vi "Dictionary.Compare.vi"(8 "error in (no error)":errorcluster, 10 "Original Data (Dictionary)":T1[](array[typedef]), 11 "Converted Data (Dictionary)":T1[](array[typedef])) -> (0 "error out":errorcluster, 3 "Not Equal?":bool)   [LabVIEW 2019, in "Conversion.lvclass"]
uses:
  Conversion.lvclass
  _OpenG.lib/numeric/numeric.llb/Random Number Within Range - I32__ogtk.vi
  Data/Typedefs/Dictionary--cluster.ctl
  Data/Data.lvclass
panel:
  out "element":string
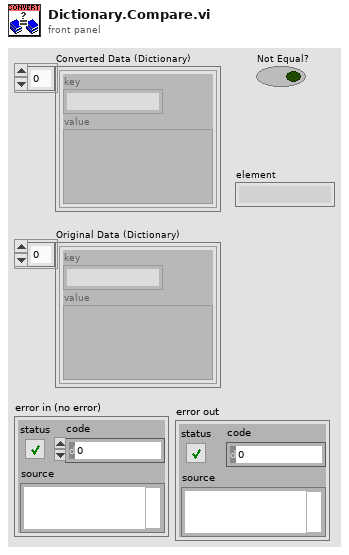
[diagram p1: front panel]
types:
  T1 = typedef "Data.lvclass/Dictionary--cluster.ctl" = cluster{"key":string, "value":variant}
  T2 = typedef "Dictionary Object RefNum__ogtk.ctl" = refnum<k1>
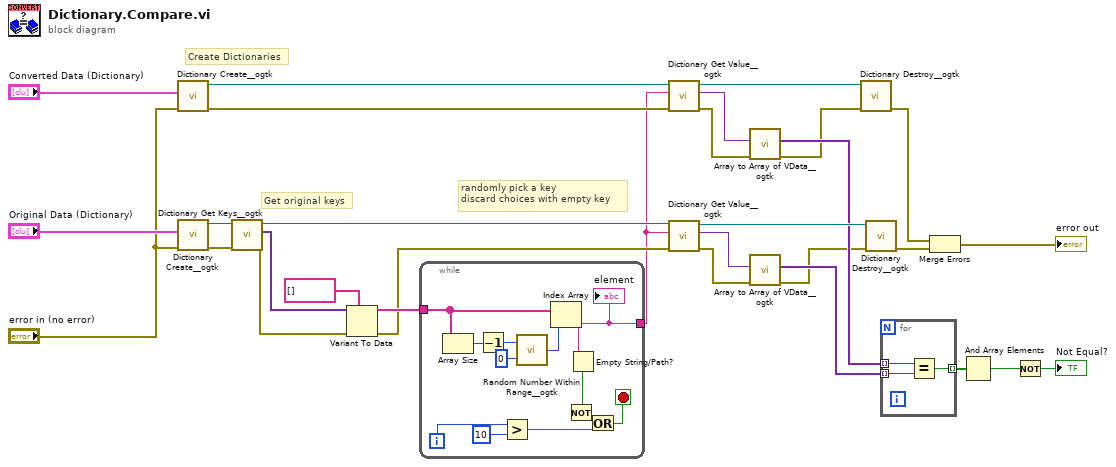
[diagram p0: block diagram]
diagram:
  # "randomly pick a key\ndiscard choices with empty key"
  # "Get original keys"
  # "Create Dictionaries"
  n1 = call "Dictionary Create__ogtk.vi"("error in (no error)"="error in (no error)", "initial dictionary (empty)"="Converted Data (Dictionary)") -> ("error out"=w18:errorcluster, "dictionary out"=w19:T2)  [unwired: 8 in]
  n2 = call "Dictionary Create__ogtk.vi"("error in (no error)"="error in (no error)", "initial dictionary (empty)"="Original Data (Dictionary)") -> ("error out"=w27:errorcluster, "dictionary out"=w28:T2)  [unwired: 8 in]
  n3 = call "Dictionary Get Keys__ogtk.vi"("error in (no error)"=w27, "dictionary"=w28) -> ("error out"=w24:errorcluster, "keys"=w23:variant[], "dictionary out"=w29:T2)  [unwired: 7 in]
  n4 = Variant To Data(error in=w24, type=string[] [], Variant=w23) -> (data=w30:string[], error out=w21:errorcluster)
  n5 = while {
    tunnel: w30 -> [w42]
    tunnel: [w37] -> w17
    i -> [w36]
    stop <- w32 stop-if-true
    n6 = Array Size(array=w42) -> (size(s)=w39:i32)
    n7 = Decrement(x=w39) -> (x-1=w38:i32)
    n8 = Greater?(x=w36, y=10) -> (0:w34:bool)
    n9 = call-poly "Random Number Within Range__ogtk.vi"("High"=w38, "Low"=0) -> ("Random Number"=w41:i32)  [unwired: 3 in]
    n10 = Index Array(array=w42, index=w41) -> (element=w37:string)
    "element" <- w37
    n11 = Empty String/Path?(string/path=w37) -> (empty?=w33:bool)
    n12 = Not(x=w33) -> (.not. x?=w31:bool)
    n13 = Or(x=w31, y=w34) -> (x .or. y?=w32:bool)
  }
  n14 = call "Dictionary Get Value__ogtk.vi"("error in"=w18, "key"=w17, "dictionary"=w19) -> ("error out"=w1:errorcluster, "value"=w8:variant, "dictionary out"=w12:T2)  [unwired: 5 in, 1 out]
  n15 = call "Dictionary Get Value__ogtk.vi"("error in"=w21, "key"=w17, "dictionary"=w29) -> ("error out"=w7:errorcluster, "value"=w2:variant, "dictionary out"=w13:T2)  [unwired: 5 in, 1 out]
  n16 = call "Array to Array of VData__ogtk.vi"("error in (no error)"=w1, "MultiD Array"=w8) -> ("error out"=w4:errorcluster, "1D Array of Variants"=w5:variant[])  [unwired: 8 in]
  n17 = call "Array to Array of VData__ogtk.vi"("error in (no error)"=w7, "MultiD Array"=w2) -> ("error out"=w3:errorcluster, "1D Array of Variants"=w6:variant[])  [unwired: 8 in]
  n18 = call "Dictionary Destroy__ogtk.vi"("error in (no error)"=w4, "dictionary"=w12) -> ("error out"=w10:errorcluster)  [unwired: 9 in]
  n19 = call "Dictionary Destroy__ogtk.vi"("error in (no error)"=w3, "dictionary"=w13) -> ("error out"=w11:errorcluster)  [unwired: 9 in]
  n20 = for {
    tunnel: w6 -> [w45] mode=indexing
    tunnel: w5 -> [w44] mode=indexing
    tunnel: [w43] -> w16 mode=indexing
    n21 = Equal?(x=w44, y=w45) -> (x = y?=w43:bool)
  }
  n22 = Merge Errors(w10, w11) -> (→"error out":errorcluster)
  n23 = And Array Elements(Boolean array=w16) -> (logical AND=w15:bool)
  n24 = Not(x=w15) -> (.not. x?=→"Not Equal?":bool)
